vi "VeristandInitialize.vi"(5 "Project File Path":path, 7 "Sequence Context":refnum<k7>, 8 "Password":string, 9 "Username":string, 10 "Visible":bool, 11 "Gateway IP Address (\"\": localhost)":string) -> (0 "error out":errorcluster, 2 "Project File Path out":path)   [LabVIEW 2015, in "MiscHelperVIs.lvlib"]
uses:
  MiscHelperVIs.lvlib
  NationalInstruments.VeriStand.ClientAPI
  <vilib>/NI Veristand/Execution/Project/NI_VS Project ExecutionAPI.lvlib
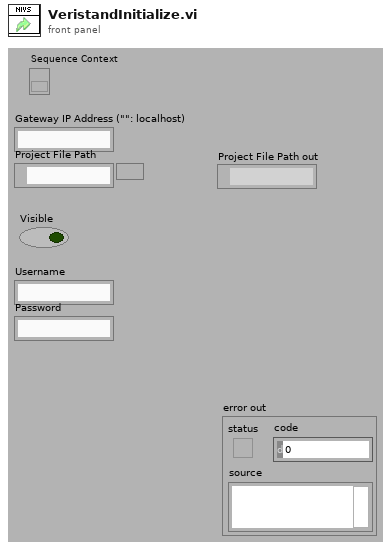
[diagram p1: front panel]
types:
  T1 = typedef "MiscHelperVIs.lvlib/VeriStand dotNet References.ctl" = cluster{"Project Ref":refnum<k24>, "Workspace Manager Ref":refnum<k24>, "Model Manager Ref":refnum<k24>, "Channel Fault Manager Ref":refnum<k24>}
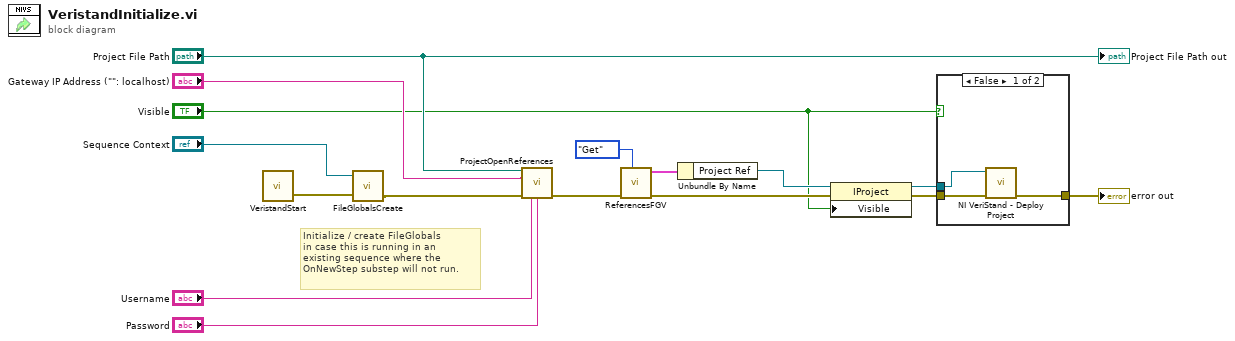
[diagram p0: block diagram]
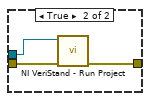
[diagram p2: hidden frame]
diagram:
  # "Initialize / create FileGlobals\nin case this is running in an \nexisting sequence where the \nOnNewStep substep will not run."
  n1 = call "VeristandStart.vi"() -> ("error out"=w16:errorcluster)  [unwired: 3 in]
  n2 = call "FileGlobalsCreate.vi"("error in (no error)"=w16, "Sequence Context"="Sequence Context") -> ("error out"=w14:errorcluster)  [unwired: 3 in]
  n3 = call "ProjectOpenReferences.vi"("Project File Path"="Project File Path", "Gateway IP Address (\"\": localhost)"="Gateway IP Address (\"\": localhost)", "error in (no error)"=w14, "Username"="Username", "Password"="Password") -> ("error out"=w9:errorcluster)  [unwired: 10 in]
  n4 = call "ReferencesFGV.vi"("Get/Set"=enum16{"Get", "Set"}."Get", "error in (no error)"=w9) -> ("error out"=w5:errorcluster, "VeriStand dotNET Refs out"=w7:T1)  [unwired: 8 in]
  n5 = Unbundle By Name(w7) -> ("Project Ref"=w6:refnum<k24>)
  n6 = property class="IProject"(reference=w6, error in=w5, "Visible"="Visible") -> (reference out=w2:refnum<k24>, error out=w3:errorcluster)
  n7 = case shown="False" "Visible" {
    tunnel: w3 -> [w19 w22]
    tunnel: w2 -> [w17 w20]
    tunnel: [w18 w21] -> w1
    frame False {
      n8 = call <vilib>:"NI VeriStand - Deploy Project.vi"("error in (no error)"=w19, "Project Ref in"=w17) -> ("error out"=w18:errorcluster)  [unwired: 8 in, 1 out]
    }
    frame True {
      n9 = call <vilib>:"NI VeriStand - Run Project.vi"("error in (no error)"=w22, "Project Ref in"=w20) -> ("error out"=w21:errorcluster)  [unwired: 8 in, 1 out]
    }
  }
  "error out" <- w1
  "Project File Path out" <- "Project File Path"
